vi "Allign FFT Frames.vi"(8 "error in (no error)":errorcluster, 10 "FFT Size":i32, 11 "FFT Frame in":refnum<class "2D Array f32.lvclass">) -> (0 "error out":errorcluster, 2 "FFT Size/2":u64, 3 "Alligned FFT Frame Out":refnum<class "2D Array f32.lvclass">)   [LabVIEW 2025, in "Signal Analysis.lvlib" / "Signal Analysis.lvclass"]
uses:
  Signal Analysis.lvclass
  <vilib>/Natan Biesmans/G2CPU GPU and CPU HPC Toolkit/G2CPU Libraries/Arrays/2DArray/f32/2D Array f32.lvclass
  6ab0c56c-33c5-4921-85f6-da3b07a79a6a.vi
  a507ae72-09cf-47cb-bf4e-c58373921f0a.vi
  1af75a38-e5b4-41cb-89d9-4bd57041f25f.vi
  f42df3b3-d3b8-4081-bb74-5b8623e75880.vi
  f7bfd20c-b87d-4f57-8e3d-07e2db968744.vi
  6ab0c56c-33c5-4921-85f6-da3b07a79a6a.vi/ab6cfe59-c8ad-4da3-839b-8d02ec9e015f.vi
  a507ae72-09cf-47cb-bf4e-c58373921f0a.vi/2e03f477-51b7-4ba0-bb4f-4f838f6557e6.vi
  a507ae72-09cf-47cb-bf4e-c58373921f0a.vi/125d45d4-836b-469d-8a4a-6adb452f866d.vi
  a507ae72-09cf-47cb-bf4e-c58373921f0a.vi/8038e9ed-2e71-4568-91ba-0d873494c5ed.vi
  1af75a38-e5b4-41cb-89d9-4bd57041f25f.vi/5793b77b-c002-4ebf-9075-685617c95341.vi
  1af75a38-e5b4-41cb-89d9-4bd57041f25f.vi/2ed3ef86-c00d-4d71-b84c-20267a6dfcf9.vi
  f42df3b3-d3b8-4081-bb74-5b8623e75880.vi/2e03f477-51b7-4ba0-bb4f-4f838f6557e6.vi
  f42df3b3-d3b8-4081-bb74-5b8623e75880.vi/125d45d4-836b-469d-8a4a-6adb452f866d.vi
  f42df3b3-d3b8-4081-bb74-5b8623e75880.vi/8038e9ed-2e71-4568-91ba-0d873494c5ed.vi
  f7bfd20c-b87d-4f57-8e3d-07e2db968744.vi/51c1d4c7-dece-4c02-9cce-b98611dadc4a.vi
  f7bfd20c-b87d-4f57-8e3d-07e2db968744.vi/3d9751b5-328d-444c-aff4-1d084998b389.vi
  6ab0c56c-33c5-4921-85f6-da3b07a79a6a.vi/ab6cfe59-c8ad-4da3-839b-8d02ec9e015f.vi/313ec8c5-c203-475c-9de0-0583f6fb8b4d.vi
  a507ae72-09cf-47cb-bf4e-c58373921f0a.vi/2e03f477-51b7-4ba0-bb4f-4f838f6557e6.vi/d8e2d9cc-c923-495e-b121-b6b84788c73f.vi
  a507ae72-09cf-47cb-bf4e-c58373921f0a.vi/2e03f477-51b7-4ba0-bb4f-4f838f6557e6.vi/345e91f0-9a5e-4de4-af9c-133346717e4a.vi
  1af75a38-e5b4-41cb-89d9-4bd57041f25f.vi/5793b77b-c002-4ebf-9075-685617c95341.vi/2c12aba4-aacf-4d7a-adbe-039f6155a93e.vi
  1af75a38-e5b4-41cb-89d9-4bd57041f25f.vi/5793b77b-c002-4ebf-9075-685617c95341.vi/f38cccb2-46f6-49f0-a8d6-9da0c88ff6f3.vi
  1af75a38-e5b4-41cb-89d9-4bd57041f25f.vi/5793b77b-c002-4ebf-9075-685617c95341.vi/bdde7ba0-fc5a-4512-a8ec-1695e5fcee25.vi
  1af75a38-e5b4-41cb-89d9-4bd57041f25f.vi/5793b77b-c002-4ebf-9075-685617c95341.vi/3e802c67-fb96-46a3-ae13-4994a8508b4f.vi
  1af75a38-e5b4-41cb-89d9-4bd57041f25f.vi/5793b77b-c002-4ebf-9075-685617c95341.vi/5a50fc67-79e7-4972-80c2-92243cd53dd4.vi
  1af75a38-e5b4-41cb-89d9-4bd57041f25f.vi/2ed3ef86-c00d-4d71-b84c-20267a6dfcf9.vi/730f6c57-5c0b-4ee9-b61e-75067b25222b.vi
  1af75a38-e5b4-41cb-89d9-4bd57041f25f.vi/2ed3ef86-c00d-4d71-b84c-20267a6dfcf9.vi/096b8799-7810-404e-baca-ba9279cec4bd.vi
  1af75a38-e5b4-41cb-89d9-4bd57041f25f.vi/2ed3ef86-c00d-4d71-b84c-20267a6dfcf9.vi/0f1a5a47-bcc5-4796-ac31-8dfcfbc0d7d1.vi
  1af75a38-e5b4-41cb-89d9-4bd57041f25f.vi/2ed3ef86-c00d-4d71-b84c-20267a6dfcf9.vi/89f12e17-3330-4b72-ad8f-8dd636660732.vi
  f42df3b3-d3b8-4081-bb74-5b8623e75880.vi/2e03f477-51b7-4ba0-bb4f-4f838f6557e6.vi/d8e2d9cc-c923-495e-b121-b6b84788c73f.vi
  f42df3b3-d3b8-4081-bb74-5b8623e75880.vi/2e03f477-51b7-4ba0-bb4f-4f838f6557e6.vi/345e91f0-9a5e-4de4-af9c-133346717e4a.vi
  1af75a38-e5b4-41cb-89d9-4bd57041f25f.vi/5793b77b-c002-4ebf-9075-685617c95341.vi/5a50fc67-79e7-4972-80c2-92243cd53dd4.vi/1b7cf390-2ae0-48f3-9bce-03c57eed6ee8.vi
  <vilib>/Natan Biesmans/G2CPU GPU and CPU HPC Toolkit/G2CPU Libraries/Arrays/1DArray/u32/1D Array u32.lvclass
  <vilib>/Natan Biesmans/G2CPU GPU and CPU HPC Toolkit/G2CPU Libraries/Arrays/1DArray/s32/1D Array s32.lvclass
  <vilib>/Natan Biesmans/G2CPU GPU and CPU HPC Toolkit/G2CPU Libraries/Arrays/1DArray/u64/1D Array u64.lvclass
  <vilib>/Natan Biesmans/G2CPU GPU and CPU HPC Toolkit/ArrayFire Driver/VIs/range.vi
  <vilib>/Natan Biesmans/G2CPU GPU and CPU HPC Toolkit/G2CPU Libraries/Arrays/Array/G2CPU Set Array Pointer.vi
  <vilib>/Natan Biesmans/G2CPU GPU and CPU HPC Toolkit/G2CPU Libraries/Arrays/Array/G2CPU Get Array Pointer.vi
  <vilib>/Natan Biesmans/G2CPU GPU and CPU HPC Toolkit/ArrayFire Driver/VIs/cast.vi
  <vilib>/Natan Biesmans/G2CPU GPU and CPU HPC Toolkit/G2CPU Libraries/Arrays/Array/G2CPU Unlock Array.vi
  <vilib>/Natan Biesmans/G2CPU GPU and CPU HPC Toolkit/G2CPU Libraries/Arrays/Array/G2CPU Release Array.vi
  <vilib>/Natan Biesmans/G2CPU GPU and CPU HPC Toolkit/ArrayFire Driver/VIs/lookup.vi
  <vilib>/Natan Biesmans/G2CPU GPU and CPU HPC Toolkit/ArrayFire Driver/VIs/Run as Multi Device.vi
  <vilib>/Natan Biesmans/G2CPU GPU and CPU HPC Toolkit/G2CPU Libraries/Manage Environment/Find AF DLL.vi
  <vilib>/Natan Biesmans/G2CPU GPU and CPU HPC Toolkit/ArrayFire Driver/subvi/Error Converter (ErrCode or Status).vi
  <vilib>/Natan Biesmans/G2CPU GPU and CPU HPC Toolkit/G2CPU Libraries/Arrays/SubVI/Lock Arrays.vi
  <vilib>/Natan Biesmans/G2CPU GPU and CPU HPC Toolkit/G2CPU Libraries/Arrays/SubVI/is 1D.vi
  <vilib>/Natan Biesmans/G2CPU GPU and CPU HPC Toolkit/ArrayFire Driver/VIs/add.vi
  <vilib>/Natan Biesmans/G2CPU GPU and CPU HPC Toolkit/ArrayFire Driver/VIs/join.vi
  <vilib>/Natan Biesmans/G2CPU GPU and CPU HPC Toolkit/G2CPU Libraries/Arrays/Array/Array Prototype.lvclass
  <vilib>/Natan Biesmans/G2CPU GPU and CPU HPC Toolkit/G2CPU Libraries/Arrays/DataTypes/I32/s32.lvclass
  <vilib>/Natan Biesmans/G2CPU GPU and CPU HPC Toolkit/G2CPU Libraries/Arrays/1DArray/1D Array Prototype.lvclass
  <vilib>/Natan Biesmans/G2CPU GPU and CPU HPC Toolkit/G2CPU Libraries/Arrays/DataTypes/U32/U32.lvclass
  Signal Analysis.lvclass/Signal Analysis.ctl
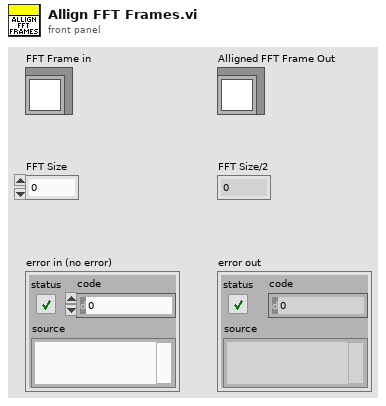
[diagram p1: front panel]
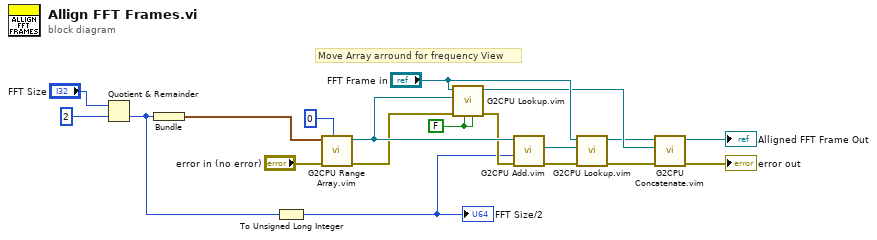
[diagram p0: block diagram]
diagram:
  w10 = FALSE ("Auto Release Array In (Enabled)")
  # "Move Array arround for frequency View"
  n1 = Quotient & Remainder(x="FFT Size", y=u64 2 ("Datatype")) -> (floor(x/y)=w14:u64)  [unwired: 1 out]
  n2 = Bundle(w14) -> (w13:cluster{u64})  [unwired: 1 in]
  n3 = To Unsigned Long Integer(number=w14) -> (unsigned 32bit integer=w1:u32)
  "FFT Size/2" <- w1
  n4 = call "G2CPU Range Array.vim"("Datatype"=u32 0, "Error in"="error in (no error)", "Size"=w13) -> ("error out"=w6:errorcluster, "Array out"=w9:refnum<class "1D Array u32.lvclass">)  [unwired: 7 in]
  n5 = call "G2CPU Lookup.vim"("Auto Release Indices (Enabled)"=w10, "Auto Release Array In (Enabled)"=w10, "error in (no error)"=w6, "Indices (1D)"=w9, "Array In"="FFT Frame in") -> ("error out"=w3:errorcluster, "Indexed Array"=w5:refnum<class "2D Array f32.lvclass">)  [unwired: 5 in]
  n6 = call "G2CPU Add.vim"("error in (no error)"=w3, "Array rhs"=w1, "Array lhs"=w9) -> ("error out"=w7:errorcluster, "Array Result"=w8:refnum<class "1D Array u32.lvclass">)  [unwired: 7 in]
  n7 = call "G2CPU Lookup.vim"("error in (no error)"=w7, "Indices (1D)"=w8, "Array In"="FFT Frame in") -> ("error out"=w2:errorcluster, "Indexed Array"=w4:refnum<class "2D Array f32.lvclass">)  [unwired: 7 in]
  n8 = call "G2CPU Concatenate.vim"("error in (no error)"=w2, "Second Array In"=w5, "First Array In"=w4) -> ("error out"=→"error out":errorcluster, "Array out"=→"Alligned FFT Frame Out":refnum<class "2D Array f32.lvclass">)  [unwired: 7 in]
